vi "fpga_Calculate Timestamp (32ch).vi"(0 "resample data and position":T1 {"frequency" format="%.59g"; "Resample position" format="%.53g"; "even-angle signal" format="%.30g"}, 5 "timestamp&count":T3 {"TAI timestamp" format="%.42g"}, 7 "muti_ch position valid?":bool, 9 "input valid":bool, 12 "ready for output":bool) -> (4 "Resample data and time":T2, 10 "output valid":bool, 14 "ready for input":bool)   [LabVIEW 2014, in "NI_EP_Resample_FPGA.lvlib"]
uses:
  <vilib>/addons/Electrical Power/PQ/Resampling/NI_EP_Resample_FPGA.lvlib
  <vilib>/addons/Electrical Power/PQ/Resampling/FPGA/subVIs/fpga_Resampled.ctl
  <vilib>/rvi/FXPMathLib/basic elements/FxpDiscreteDelay/XNode/nifxpmath_DiscreteDelay.xnode
  <vilib>/rvi/FXPMathLib/FxpSub/XNode/nifxpmath_Sub.xnode
  <vilib>/rvi/FXPMathLib/FxpMul/XNode/nifxpmath_Multiplier.xnode
  <vilib>/rvi/FXPMathLib/sim/FxpSim.dll
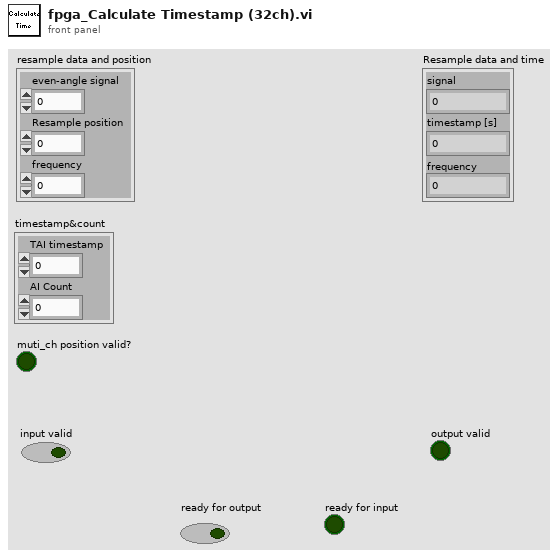
[diagram p1: front panel]
types:
  T1 = cluster{"even-angle signal":fxp<+/-,32,3>, "Resample position":fxp<+,64,16>, "frequency":fxp<+,32,8>}
  T2 = typedef "NI_EP_Resample_FPGA.lvlib/fpga_Resampled.ctl" = cluster{"signal":fxp<+/-,32,3>, "timestamp [s]":fxp<+,64,32>, "frequency":fxp<+,32,8>}
  T3 = cluster{"TAI timestamp":fxp<+,64,32>, "AI Count":u16}
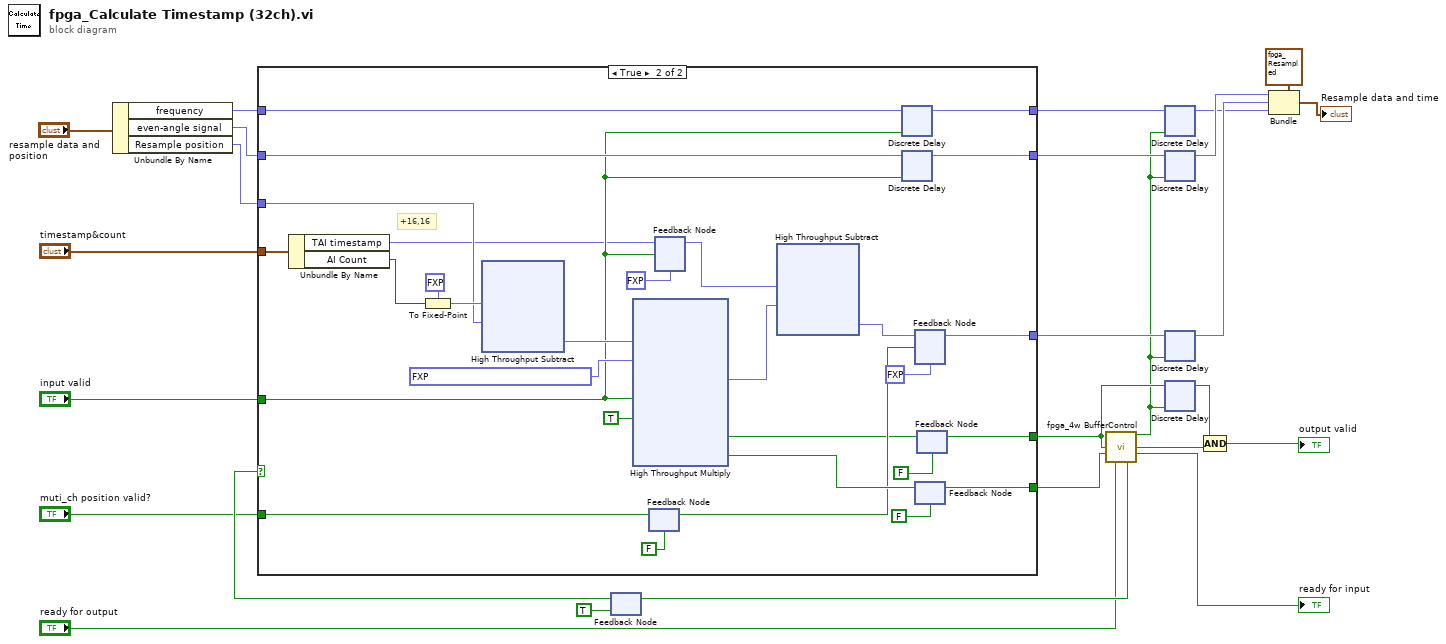
[diagram p0: block diagram]
diagram:
  n1 = Unbundle By Name("resample data and position") -> ("frequency"=w5:fxp<+,32,8>, "even-angle signal"=w4:fxp<+/-,32,3>, "Resample position"=w3:fxp<+,64,16>)
  n2 = feedback #1(TRUE ("logic enable")) -> (w24:bool)
  n3 = case shown="True" w24 {
    tunnel: "timestamp&count" -> [_ w32]
    tunnel: w4 -> [_ w39]
    tunnel: w3 -> [_ w34]
    tunnel: w5 -> [_ w41]
    tunnel: "input valid" -> [_ w30]
    tunnel: "muti_ch position valid?" -> [_ w47]
    tunnel: [_ w46] -> w11
    tunnel: [_ w43] -> w15
    tunnel: [_ w40] -> w14
    tunnel: [_ w38] -> w13
    tunnel: [_ w42] -> w12
    frame False {
    }
    frame True {
      # "+16,16"
      n4 = Unbundle By Name(w32) -> ("TAI timestamp"=w28:fxp<+,64,32>, "AI Count"=w31:u16)
      n5 = To Fixed-Point(fixed-point type=fxp<+,16,16> 0.0, number=w31) -> (fixed-point=w54:fxp<+,16,16>)
      n6 = xnode "High Throughput Subtract"("x"=w54, "y"=w34) -> ("x-y"=w36:fxp<+,32,16>)
      n7 = xnode ("High Throughput Multiply")("x"=w36, "y"=fxp<+,16,-15> 2.00001522898674e-05 ("Numeric"), "input valid"=w30, "ready for output (T)"=TRUE) -> ("x*y"=w52:fxp<+,64,32>, "output valid"=w29:bool, "ready for input"=w44:bool)
      n8 = feedback #2(FALSE ("muti_ch position valid?")) -> (w35:bool)
      n9 = feedback-in #2(w47) -> ()
      n10 = feedback #3(fxp<+,64,32> 0.0 ("TAI timestamp")) -> (w27:fxp<+,64,32>)
      n11 = feedback-in #3(w28, w30) -> ()
      n12 = xnode "High Throughput Subtract"("x"=w27, "y"=w52) -> ("x-y"=w51:fxp<+,64,32>)
      n13 = xnode ("Discrete Delay")("D"=w41, "enable"=w30) -> ("Q"=w40:fxp<+,32,8>)
      n14 = xnode ("Discrete Delay")("D"=w39, "enable"=w30) -> ("Q"=w38:fxp<+/-,32,3>)
      n15 = feedback #4(fxp<+,64,32> 0.0 ("x-y")) -> (w42:fxp<+,64,32>)
      n16 = feedback-in #4(w51, w35) -> ()
      n17 = feedback #5(FALSE ("output valid")) -> (w43:bool)
      n18 = feedback-in #5(w44) -> ()
      n19 = feedback #6(FALSE ("output valid")) -> (w46:bool)
      n20 = feedback-in #6(w29) -> ()
    }
  }
  n21 = call <vilib>:"fpga_4w BufferControl.vi"("DR"=w11, "RFI"=w15, "RFO"="ready for output") -> ("buff enable"=w1:bool, "output valid"=w21:bool, "ready for input"=→"ready for input":bool, "logic enable"=w26:bool)  [unwired: 9 in]
  n22 = feedback-in #1(w26) -> ()
  n23 = xnode ("Discrete Delay")("D"=w14, "enable"=w1) -> ("Q"=w8:fxp<+,32,8>)
  n24 = xnode ("Discrete Delay")("D"=w13, "enable"=w1) -> ("Q"=w10:fxp<+/-,32,3>)
  n25 = xnode ("Discrete Delay")("D"=w12, "enable"=w1) -> ("Q"=w9:fxp<+,64,32>)
  n26 = xnode ("Discrete Delay")("D"=w11, "enable"=w1) -> ("Q"=w23:bool)
  n27 = Compound Arithmetic op=AND(w23, w21) -> (→"output valid":bool)
  n28 = Bundle(cluster=T2 {"signal"=0.0, "timestamp [s]"=0.0, "frequency"=0.0} ("Resample data and time"), "signal"=w10, "timestamp [s]"=w9, "frequency"=w8) -> (→"Resample data and time":T2)
